vi "PreviewNextOperation.vi"(6 "Timeout in ms (-1)":i32, 8 "error in (no error)":errorcluster, 11 "SMP in":refnum<class "SMP.lvclass">) -> (0 "error out":errorcluster, 1 "Previous data":variant, 2 "Operation":T1, 3 "SMP out":refnum<class "SMP.lvclass">, 4 "Timed out?":bool, 5 "Pipe operation?":bool)   [LabVIEW 2013, in "SMP.lvclass"]
doc: "Previews the operation from the front of the operations queue of the SMP object without actually removing it from the queue.\n\n<b>Timeout: </b>A timeout for the preview operation. Default is -1 (never time out).\n\n<b>Pipe operation: </b>TRUE if the previewed operation is part of a pipe. FALSE otherwise.\n\n<b>Operation: </b>The previewed operation. This can be either an individual operation or an operation which is part of a pipe.\n\n<b>Previous data: </b>Data which was produced by the previous operation in the queue. This must be explicitly set using the function SetPreviousData, after the previous operation has completed.\n\n<b>Timed out: </b>TRUE if the previewed operation timed out. FALSE otherwise."
uses:
  SMP.lvclass
  Data types/operation.ctl
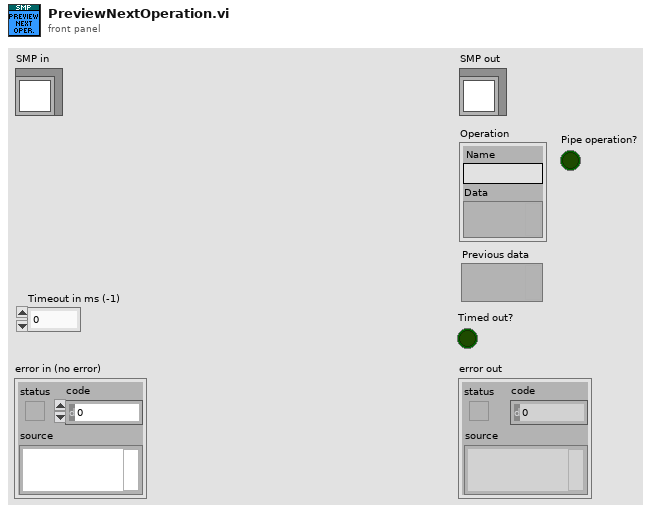
[diagram p1: front panel]
types:
  T1 = typedef "SMP.lvclass/operation.ctl" = cluster{"Name":string, "Data":variant}
  T2 = typedef "Pipe and Filter.lvclass/classData.ctl" = cluster{"Q ref":refnum<queue>, "Previous data":variant, "Current pipe":T3[]}
  T3 = typedef "Pipe and Filter.lvclass/operation.ctl" = cluster{"Name":string, "Data":variant}
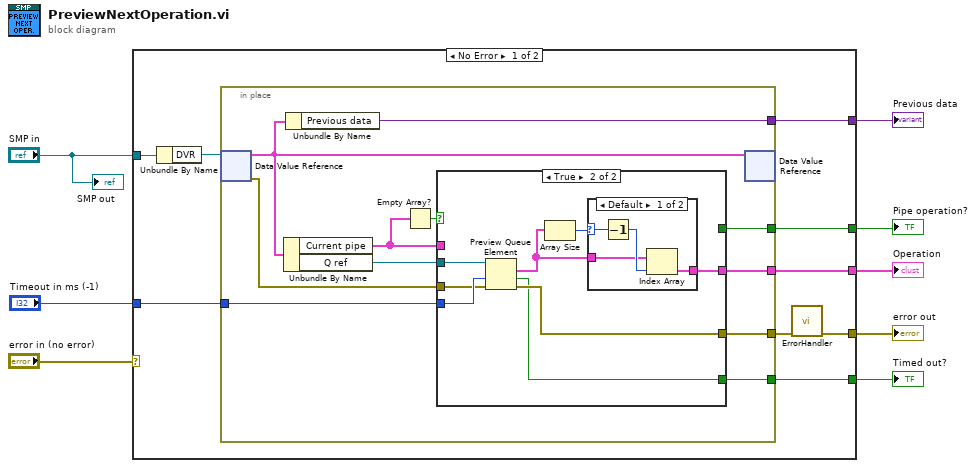
[diagram p0: block diagram]
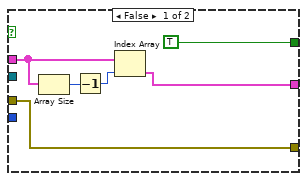
[diagram p2: hidden frame]
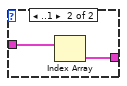
[diagram p3: hidden frame]
diagram:
  n1 = case shown="No Error" "error in (no error)" {
    selector: "error in (no error)" -> [_ w49]
    tunnel: [w14 w49] -> w7
    tunnel: "SMP in" -> [w16 _]
    tunnel: "Timeout in ms (-1)" -> [w13 _]
    tunnel: [w12 _] -> w4
    tunnel: [w11 _] -> w3
    tunnel: [w10 _] -> w2
    tunnel: [w9 _] -> w1
    frame No Error {
      n2 = Unbundle By Name(w16) -> ("DVR"=w17:refnum<data-value>)
      n3 = in-place {
        in-place-border: [w26] -> w15
        in-place-border: w13 -> [w28]
        in-place-border: [w23] -> w12
        in-place-border: [w22] -> w11
        in-place-border: [w21] -> w10
        in-place-border: [w20] -> w9
        n4 = in-place-dvr #1(w17) -> (w18:T2, w27:errorcluster)
        n5 = Unbundle By Name(w18) -> ("Current pipe"=w19:T3[], "Q ref"=w25:refnum<queue>)
        n6 = Unbundle By Name(w18) -> ("Previous data"=w23:variant)
        n7 = Empty Array?(array=w19) -> (empty?=w24:bool)
        n8 = case shown="True" w24 {
          tunnel: w28 -> [_ w42]
          tunnel: w27 -> [w34 w41]
          tunnel: [w34 w40] -> w26
          tunnel: w25 -> [_ w39]
          tunnel: [w29 w36] -> w22
          tunnel: [TRUE _] -> w21
          tunnel: [_ w35] -> w20
          tunnel: w19 -> [w32 _]
          frame False {
            n9 = Array Size(array=w32) -> (size(s)=w31:i32)
            n10 = Decrement(x=w31) -> (x-1=w30:i32)
            n11 = Index Array(array=w32, index=w30) -> (element=w29:T3)
          }
          frame True {
            n12 = Preview Queue Element(queue=w39, timeout in ms (-1)=w42, error in (no error)=w41) -> (element=w37:T3[], timed out?=w35:bool, error out=w40:errorcluster)  [unwired: 1 out]
            n13 = Array Size(array=w37) -> (size(s)=w38:i32)
            n14 = case shown="Default" w38 {
              selector: w38 -> [w44 _]
              tunnel: w37 -> [w45 w48]
              tunnel: [w43 w47] -> w36
              frame Default {
                n15 = Decrement(x=w44) -> (x-1=w46:i32)
                n16 = Index Array(array=w45, index=w46) -> (element=w43:T3)
              }
              frame ..1 {
                n17 = Index Array(array=w48) -> (element=w47:T3)  [unwired: 1 in]
              }
            }
          }
        }
        n18 = in-place-dvr #1(w18) -> ()  [unwired: 2 out]
      }
      n19 = call "ErrorHandler.vi"("error in (no error)"=w15) -> ("error out"=w14:errorcluster)  [unwired: 9 in, 1 out]
    }
    frame Error {
    }
  }
  "error out" <- w7
  "Previous data" <- w4
  "Operation" <- w3
  "Pipe operation?" <- w2
  "Timed out?" <- w1
  "SMP out" <- "SMP in"
